vi "GetXL_WorkSheetsNum.vi"(8 "error in (no error)":errorcluster, 11 "Refnum Cluster In":T1) -> (0 "error out":errorcluster, 2 "size(s)":i32, 3 "Refnum Cluster In":T1)   [LabVIEW 2017, in "excel_configuration.lvlib"]
doc: "Returns the number of worksheets in the open workbook."
uses:
  excel_configuration.lvlib
  574ec8ed-b0f7-487c-a4da-101a78198ecc.vi
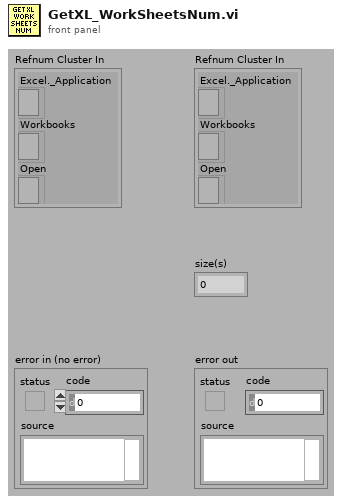
[diagram p1: front panel]
types:
  T1 = cluster{"Excel._Application":refnum<k7>, "Workbooks":refnum<k7>, "Open":refnum<k7>}
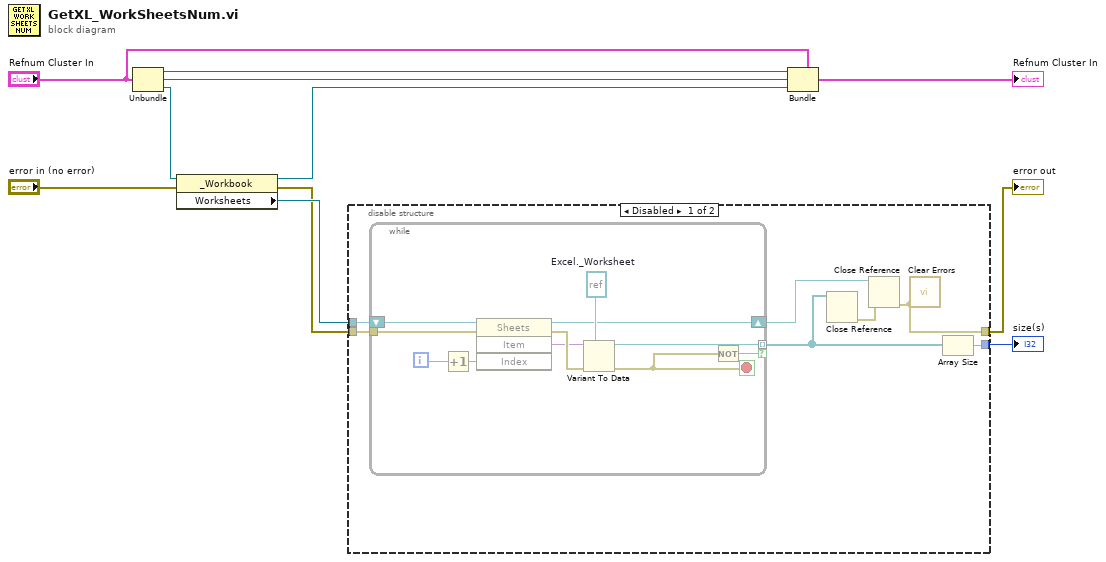
[diagram p0: block diagram]
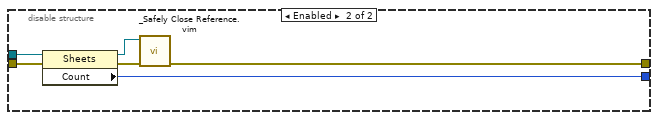
[diagram p2: hidden frame]
diagram:
  n1 = Unbundle("Refnum Cluster In") -> ("Excel._Application"=w9:refnum<k7>, "Workbooks"=w10:refnum<k7>, "Open"=w8:refnum<k7>)
  n2 = property class="_Workbook"(reference=w8, error in="error in (no error)") -> (reference out=w11:refnum<k7>, error out=w3:errorcluster, "Worksheets"=w4:refnum<k7>)
  n3 = disable-structure shown="Disabled" {
    disable-tunnel: w4 -> [w18 w35]
    disable-tunnel: w3 -> [w17 w34]
    disable-tunnel: [w16 w33] -> w2
    disable-tunnel: [w12 w30] -> w1
    frame Disabled {
      n4 = while {
        tunnel: w17 -> [w28]
        tunnel: [w22] -> w15 mode=indexing if=w20
        shift-right: [w19] -> w14
        shift-left: w18 -> [w25]
        i -> [w24]
        stop <- w21 stop-if-true
        w27 = refnum<k7> refnum  # Excel._Worksheet
        n5 = Increment(x=w24) -> (x+1=w23:i32)
        n6 = invoke class="Sheets" method="Item"(reference=w25, error in=w28, "Index"=w23) -> (reference out=w19:refnum<k7>, error out=w29:errorcluster, "Item"=w26:variant)  [unwired: 1 in, 1 out]
        n7 = Variant To Data(error in=w29, type=w27, Variant=w26) -> (data=w22:refnum<k7>, error out=w21:errorcluster)
        n8 = Not(x=w21) -> (.not. x?=w20:bool)
      }
      n9 = Close Reference(reference=w15) -> (error out=w13:errorcluster)  [unwired: 1 in]
      n10 = Close Reference(reference=w14, error in (no error)=w13) -> (error out=w12:errorcluster)
      n11 = call <vilib>:"Clear Errors.vi"("error in (no error)"=w12) -> ()  [unwired: 5 in, 2 out]
      n12 = Array Size(array=w15) -> (size(s)=w16:i32)
    }
    frame Enabled {
      n13 = property class="Sheets"(reference=w35, error in=w34) -> (reference out=w31:refnum<k7>, error out=w32:errorcluster, "Count"=w33:i32)
      n14 = call "_Safely Close Reference.vim"("error in (no error)"=w32, "Automation Refnum in"=w31) -> ("error out"=w30:errorcluster)  [unwired: 9 in]
    }
  }
  "error out" <- w1
  "size(s)" <- w2
  n15 = Bundle(cluster="Refnum Cluster In", "Excel._Application"=w9, "Workbooks"=w10, "Open"=w11) -> (→"Refnum Cluster In":T1)
